vi "Generate PPS_cRIO9039(Host).vi"() -> ()   [LabVIEW 2016]
uses:
  <vilib>/userdefined/High Color/nirio_resource_hc.ctl
  <vilib>/FPGAPlugInAG/cRIO-9039 (Sync)/niLvFpga_Open_cRIO-9039 (Sync).vi
  <vilib>/rvi/interface/common/dynamic/niFpgaDynamicAddResources.vi
  <vilib>/FPGAPlugInAG/Dynamic/niLvFpga_Run_Dynamic.vi
  <vilib>/Utility/error.llb/Error Cluster From Error Code.vi
  <vilib>/rvi/errors/niLvFpgaAdjustHostInterfaceError.vi
  <vilib>/FPGAPlugInAG/Dynamic/niLvFpga_Close_Dynamic.vi
  <vilib>/rvi/interface/nirviOpenFPGA/nirviOpenFPGA.xnode
  FPGA Bitfiles/8021ASPXIe_FPGATarget2_GeneratePPS-cRIO_4wTwTUP0plA.lvbitx
  Generate PPS-cRIO9039.vi
  <vilib>/rvi/interface/nirviMethod/nirviMethod.xnode
  <vilib>/rvi/interface/nirviReadWriteControl/nirviReadWriteControl.xnode
  <vilib>/rvi/interface/nirviCloseFPGA/nirviCloseFPGA.xnode
  <vilib>/rvi/interface/Simulation/niFpgaSimulationCallBeginRW.vi
  NiFpgaLv.dll
panel:
  out "Current Time":u64
  out "Time Synchronization Fault":bool
  out "Time Source":enum8{"None", "System", "External"}(ring)
  out "FPGA Time":timestamp
  out "Offset from Time Reference":i32
  out "Offset from Time Reference Valid":bool
  out "RT Time":timestamp
  in  "PPS Duration(Ticks)":u64=40000000 format="%.0p"
  out "error out":errorcluster
  in  "stop":bool
  in  "Resource  Name":T1="RIO0"
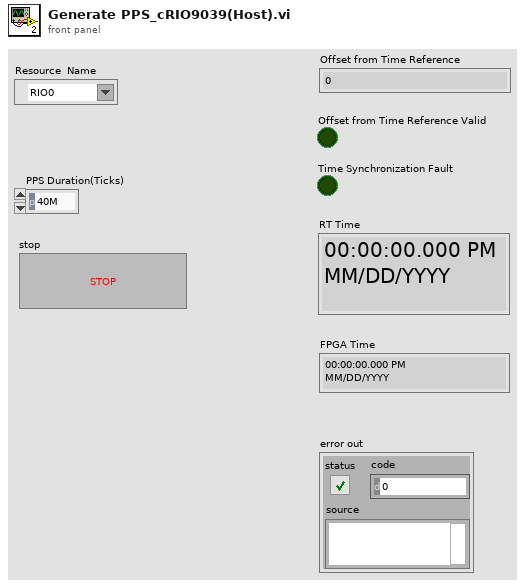
[diagram p1: front panel]
types:
  T1 = typedef "nirio_resource_hc.ctl" = tag
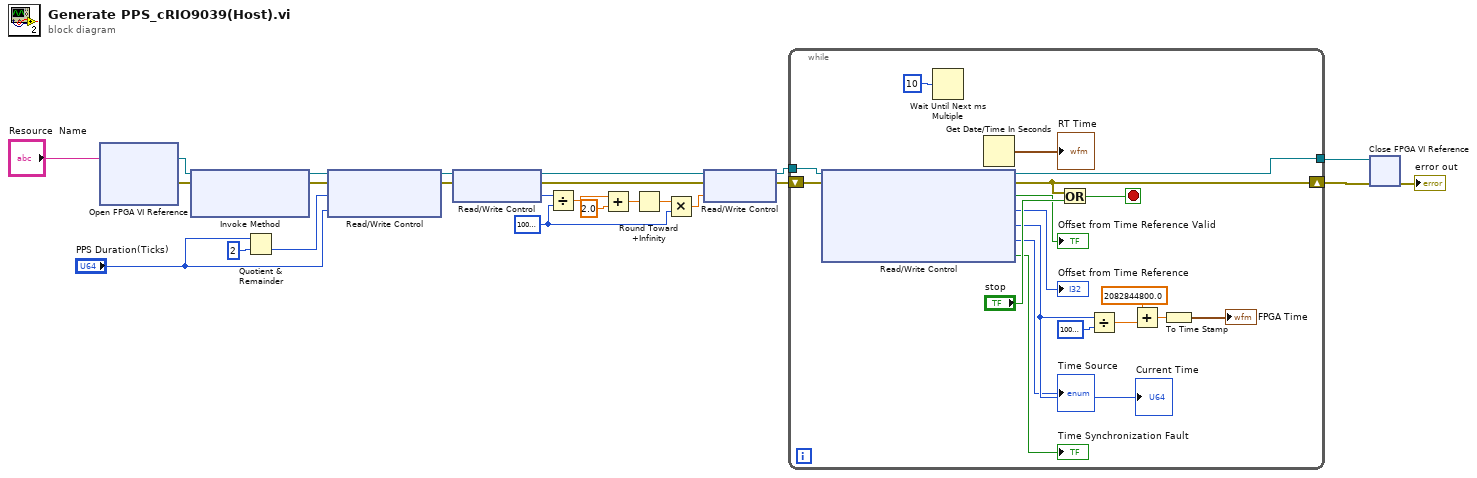
[diagram p0: block diagram]
diagram:
  w15 = u64 1000000000 ("y")
  n1 = xnode "Open FPGA VI Reference"("resource name"="Resource  Name") -> ("FPGA VI Reference Out"=w23:refnum<k20>, "error out"=w22:errorcluster)  [unwired: 1 in]
  n2 = xnode "Invoke Method"("FPGA VI Reference In"=w23, "error in"=w22) -> ("FPGA VI Reference Out"=w6:refnum<k20>, "error out"=w5:errorcluster)  [unwired: 1 in]
  n3 = Quotient & Remainder(x="PPS Duration(Ticks)", y=u64 2) -> (floor(x/y)=w2:u64)  [unwired: 1 out]
  n4 = xnode "Read/Write Control"("FPGA VI Reference In"=w6, "error in"=w5, "PulseWidth(Ticks)"=w2, "Tx Pulse Ticks"="PPS Duration(Ticks)") -> ("FPGA VI Reference Out"=w8:refnum<k20>, "error out"=w7:errorcluster)
  n5 = xnode "Read/Write Control"("FPGA VI Reference In"=w8, "error in"=w7) -> ("FPGA VI Reference Out"=w21:refnum<k20>, "error out"=w20:errorcluster, "Current Time"=w19:u64)
  n6 = Divide(x=w19, y=w15) -> (x/y=w1:dbl)
  n7 = Add(x=w1, y=2.0) -> (x+y=w17:dbl)
  n8 = Round Toward +Infinity(x=w17) -> (ceil(x): smallest int >= x=w16:dbl)
  n9 = Multiply(x=w16, y=w15) -> (x*y=w14:dbl)
  n10 = xnode "Read/Write Control"("FPGA VI Reference In"=w21, "error in"=w20, "Start Time"=w14) -> ("FPGA VI Reference Out"=w13:refnum<k20>, "error out"=w12:errorcluster)
  n11 = while {
    tunnel: w13 -> [w38]
    tunnel: [w36] -> w11
    shift-right: [w35] -> w10
    shift-left: w12 -> [w37]
    stop <- w41 stop-if-true
    n12 = xnode "Read/Write Control"("FPGA VI Reference In"=w38, "error in"=w37) -> ("FPGA VI Reference Out"=w36:refnum<k20>, "error out"=w35:errorcluster, "Offset from Time Reference Valid"=→"Offset from Time Reference Valid":bool, "Offset from Time Reference"=→"Offset from Time Reference":i32, "Current Time"=w32:u64, "Time Source"=→"Time Source":enum8{"None", "System", "External"}, "Time Synchronization Fault"=→"Time Synchronization Fault":bool)
    "Current Time" <- w32
    n13 = Wait Until Next ms Multiple(millisecond multiple=u32 10) -> ()  [unwired: 1 out]
    n14 = Get Date/Time In Seconds() -> (seconds since 1Jan1904=→"RT Time":timestamp)
    n15 = Or(x=w35, y="stop") -> (x .or. y?=w41:bool)
    n16 = Divide(x=w32, y=u64 1000000000) -> (x/y=w27:dbl)
    n17 = Add(x=2082844800.0, y=w27) -> (x+y=w26:dbl)
    n18 = To Time Stamp(1:w26) -> (0:→"FPGA Time":timestamp)
  }
  n19 = xnode "Close FPGA VI Reference"("FPGA VI Reference In"=w11, "error in"=w10) -> ("error out"=→"error out":errorcluster)
